vi "(SubVI) DownSampling Moving Filtered Data_YCC.vi"(4 "data# reduce factor":i32, 5 "Moving Filtered QPD data":dbl[](array[numeric]), 6 "Moving Filtered Stage data":dbl[](array[numeric])) -> (1 "DownSampling QPD":dbl[](array[numeric]), 2 "DownSampling Stage":dbl[](array[numeric]))   [LabVIEW 2014]
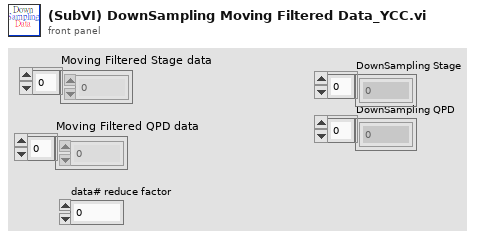
[diagram p1: front panel]
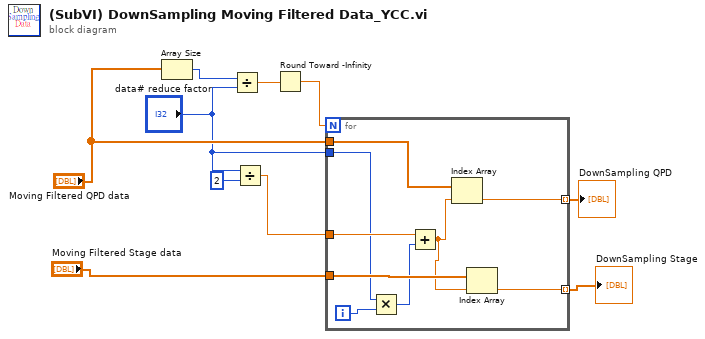
[diagram p0: block diagram]
diagram:
  n1 = Array Size(array="Moving Filtered QPD data") -> (size(s)=w10:i32)
  n2 = Divide(x=w10, y="data# reduce factor") -> (x/y=w9:dbl)
  n3 = Divide(x="data# reduce factor", y=2) -> (x/y=w4:dbl)
  n4 = Round Toward -Infinity(1:w9) -> (0:w8:dbl)
  n5 = for {
    N: w8 -> [_]
    tunnel: "Moving Filtered QPD data" -> [w19]
    tunnel: "Moving Filtered Stage data" -> [w18]
    tunnel: w4 -> [w16]
    tunnel: "data# reduce factor" -> [w15]
    tunnel: [w12] -> w2 mode=indexing
    tunnel: [w11] -> w1 mode=indexing
    i -> [w17]
    n6 = Multiply(x=w15, y=w17) -> (x*y=w14:i32)
    n7 = Add(x=w16, y=w14) -> (x+y=w13:dbl)
    n8 = Index Array(array=w19, index=w13) -> (element=w12:dbl)
    n9 = Index Array(array=w18, index=w13) -> (element=w11:dbl)
  }
  "DownSampling QPD" <- w2
  "DownSampling Stage" <- w1
